vi "8通道控制.vi"() -> ()   [LabVIEW 2010]
uses:
  <vilib>/DAQmx/read.llb/DAQmx Read (Analog 2D DBL NChan NSamp).vi
  <vilib>/DAQmx/read.llb/DAQmx Read (Analog 1D DBL NChan 1Samp).vi
  <vilib>/DAQmx/write.llb/DAQmx Write (Analog 1D DBL NChan 1Samp).vi
  <vilib>/daqmx/miscellaneous.llb/DAQmx Fill In Error Info.vi
panel:
  out "AO overload":bool[](array[boolean])
  in  "啟用控制":bool
  out "速度+加速度":T1(graph)
  out "加速度訊號":T1(graph)
  in  "Kp":dbl[](array[numeric])=[0.0, 0.0, 0.0, 0.0, 0.0, 0.0, 0.0, 0.0]
  in  "Ki":dbl[](array[numeric])=[-500.0, -500.0, -500.0, -500.0, -80.0, -80.0, -80.0, -80.0]
  out "取樣時間誤差(%)":dbl
  out "初始化 input":dbl[][](graph)
  out "速度訊號":T1(graph)
  out "迴圈時間(ms)":dbl
  in  "stop":bool
  out "error out":errorcluster
  in  "ÂoDC®É¶¡(s)":dbl=1.0
  in  "取樣頻率(Hz)":dbl=2000.0
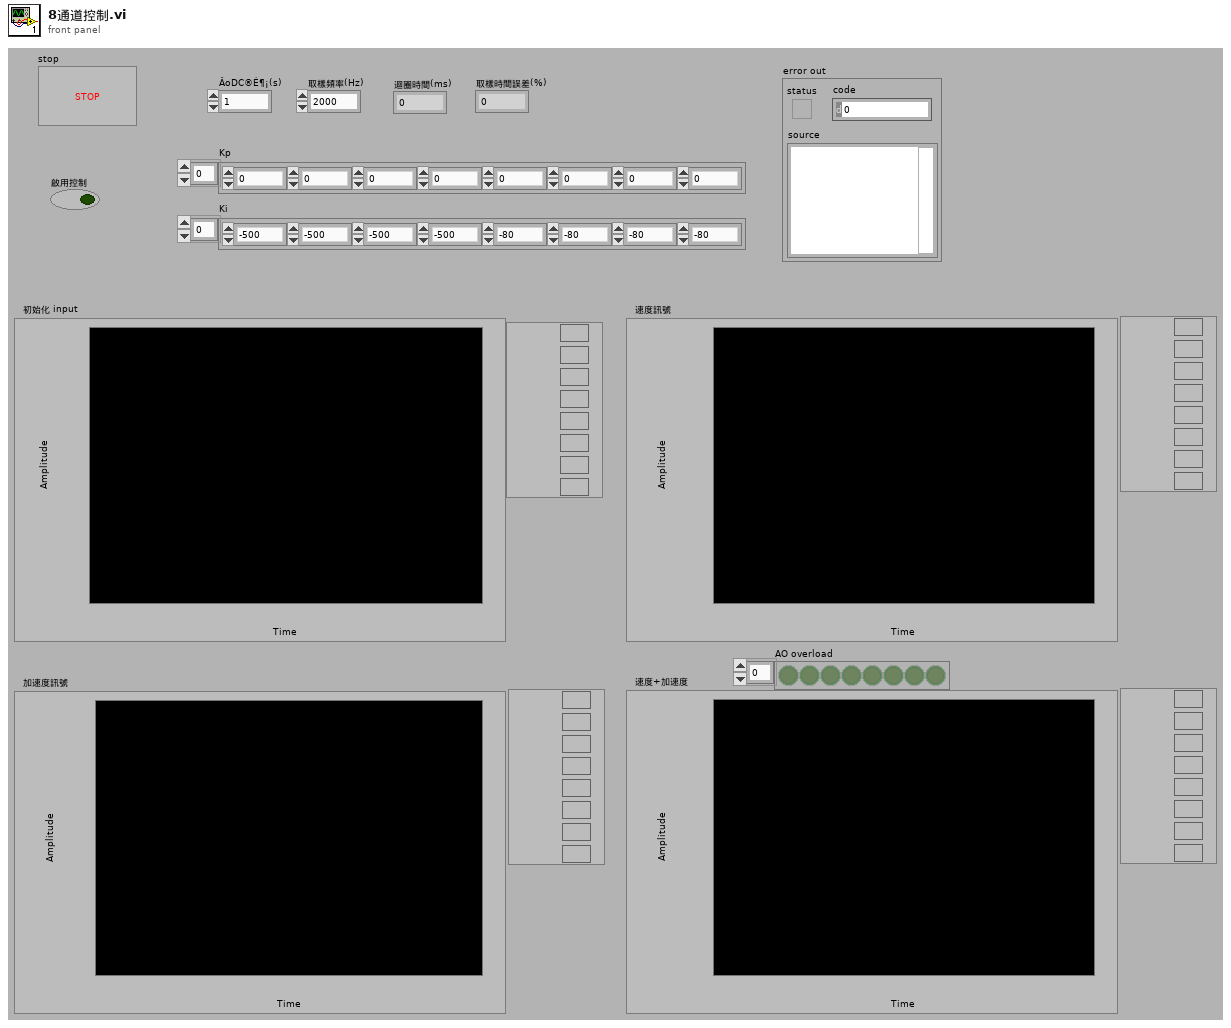
[diagram p1: front panel]
types:
  T1 = cluster{"DC Filter out[0]":dbl, "DC Filter out[1]":dbl, "DC Filter out[2]":dbl, "DC Filter out[3]":dbl, "DC Filter out[4]":dbl, "DC Filter out[5]":dbl, "DC Filter out[6]":dbl, "DC Filter out[7]":dbl}
  T2 = cluster{"[0]":dbl, "[1]":dbl, "[2]":dbl, "[3]":dbl, "[4]":dbl, "[5]":dbl, "[6]":dbl, "[7]":dbl}
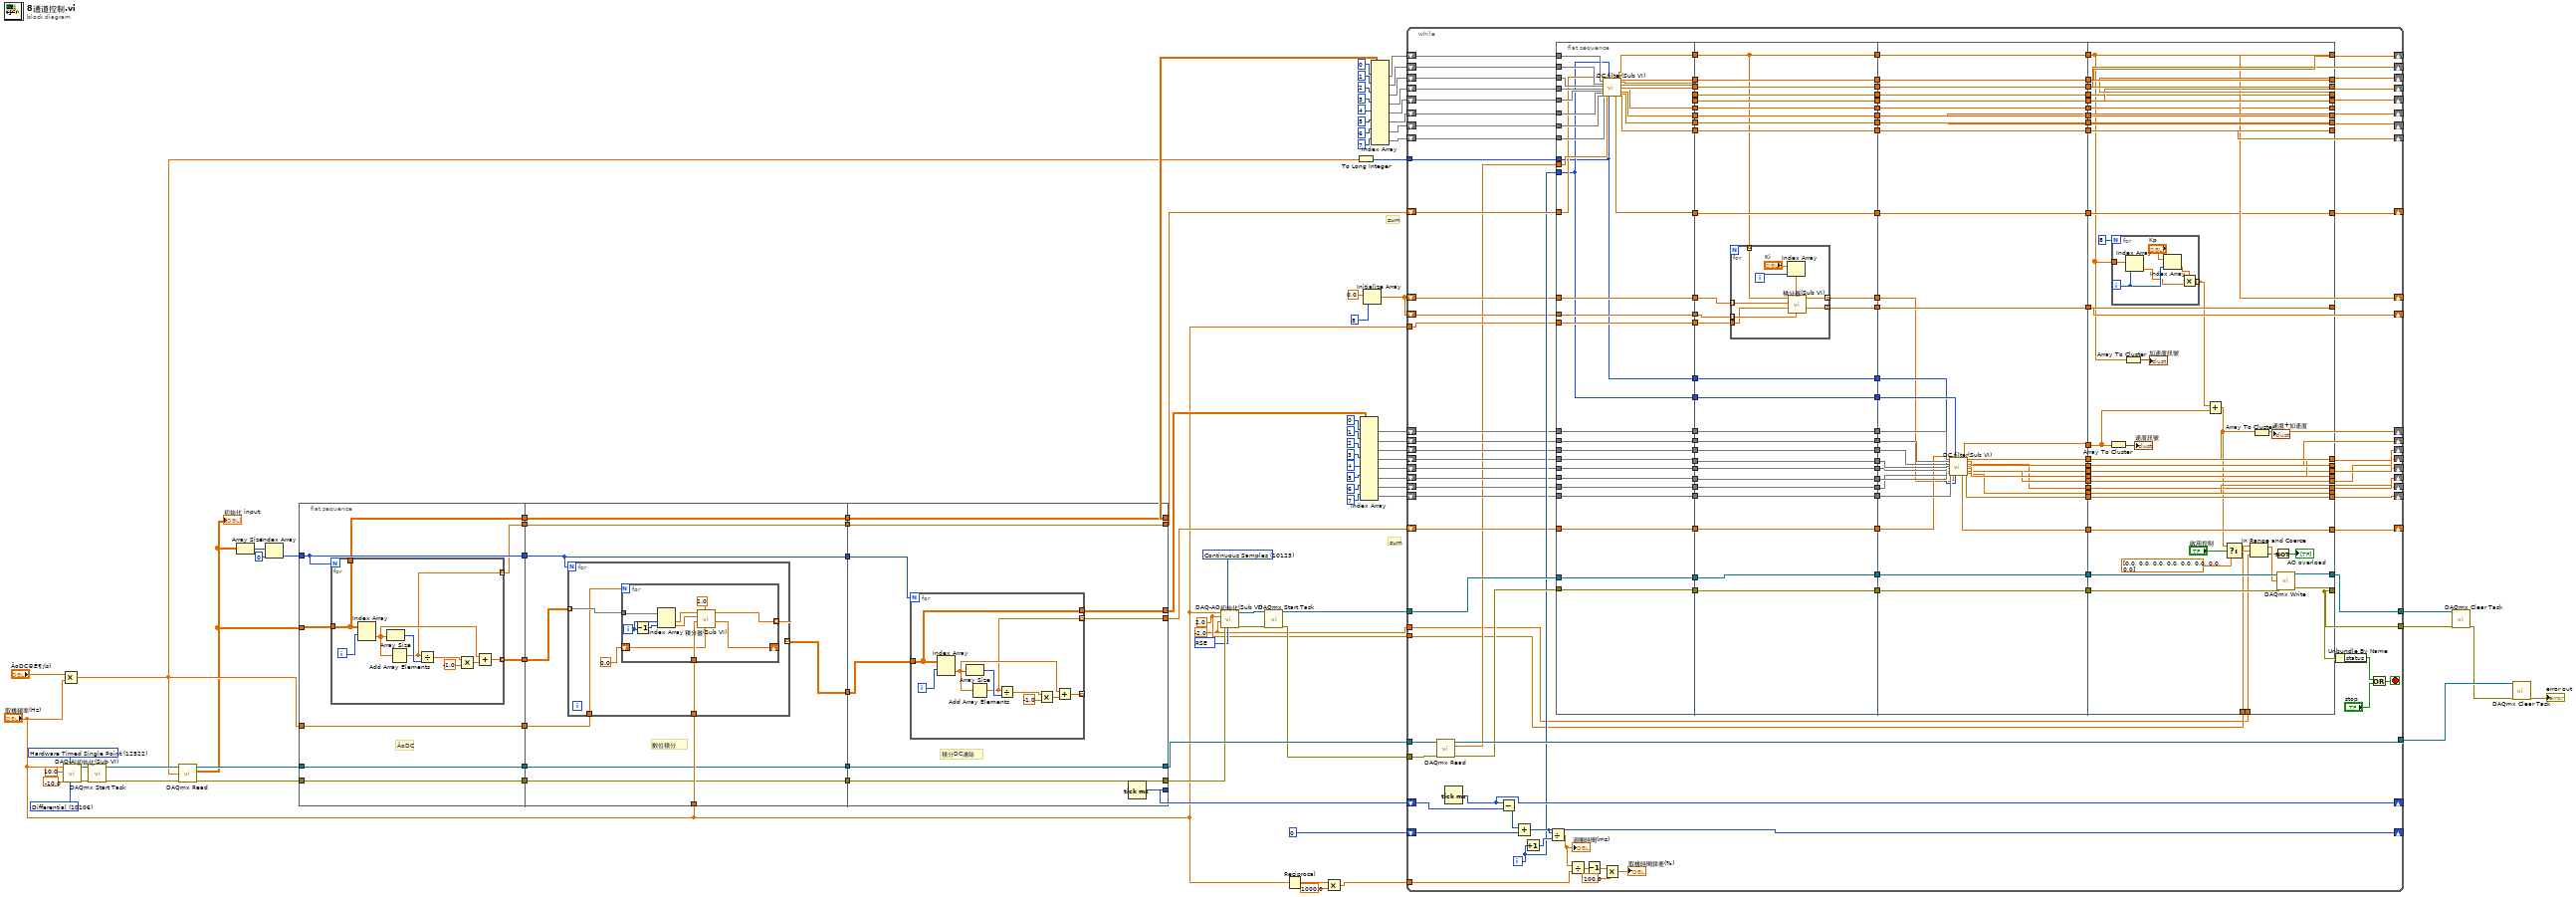
[diagram p0: block diagram]
diagram:
  w7 = 10106 items=["default"=-1, "RSE"=10083, "NRSE"=10078, "Differential"=10106, "Pseudodifferential"=12529] ("input terminal configuration")
  w10 = 10083 items=["Default"=-1, "RSE"=10083, "Differential"=10106, "Pseudodifferential"=12529] ("output terminal configuration")
  w54 = 10123 items=["Finite Samples"=10178, "Continuous Samples"=10123, "Hardware Timed Single Point"=12522] ("sample mode")
  w55 = 12522 items=["Finite Samples"=10178, "Continuous Samples"=10123, "Hardware Timed Single Point"=12522] ("sample mode")
  w1 = -2.0 ("minimum value")
  w2 = 2.0 ("maximum value")
  # "sum"
  # "sum"
  n1 = Multiply(x="ÂoDC®É¶¡(s)", y="取樣頻率(Hz)") -> (x*y=w13:dbl)
  n2 = call "DAQ-AI初始化(Sub VI).vi"("input terminal configuration"=w7, "sample mode"=w55, "minimum value"=-10.0, "maximum value"=10.0, "取樣頻率(Hz)"="取樣頻率(Hz)") -> ("error out"=w87:errorcluster, "task out"=w88:refnum<k21>)  [unwired: 5 in]
  n3 = call <vilib>:"DAQmx Start Task.vi"("task/channels in"=w88, "error in"=w87) -> ("task out"=w90:refnum<k21>, "error out"=w89:errorcluster)  [unwired: 12 in]
  n4 = call-poly <vilib>:"DAQmx Read.vi"("task/channels in"=w90, "number of samples per channel"=w13, "error in"=w89) -> ("task out"=w73:refnum<k21>, "data"=w11:dbl[][], "error out"=w76:errorcluster)  [unwired: 10 in]
  "初始化 input" <- w11
  n5 = Array Size(array=w11) -> (size(s)=w85:i32[])
  n6 = Index Array(array=w85, index=0) -> (element=w83:i32)
  n7 = flat-sequence {
    tunnel: w11 -> [w98]
    tunnel: w83 -> [w96]
    tunnel: [w97] -> w82
    tunnel: [w96] -> w80
    tunnel: w73 -> [w95]
    tunnel: [w95] -> w78
    tunnel: w76 -> [w94]
    tunnel: [w94] -> w75
    tunnel: [w93] -> w70
    tunnel: w13 -> [w93]
    tunnel: [w92] -> w60
    tunnel: [w91] -> w58
    tunnel: w82 -> [w116]
    tunnel: [w115] -> w81
    tunnel: w80 -> [w113]
    tunnel: "取樣頻率(Hz)" -> [w114]
    tunnel: [w113] -> w79
    tunnel: w78 -> [w112]
    tunnel: [w112] -> w77
    tunnel: w75 -> [w111]
    tunnel: [w111] -> w74
    tunnel: w70 -> [w110]
    tunnel: w60 -> [w109]
    tunnel: [w109] -> w59
    tunnel: w58 -> [w108]
    tunnel: [w108] -> w57
    tunnel: w81 -> [w140]
    tunnel: w79 -> [w139]
    tunnel: w77 -> [w138]
    tunnel: w74 -> [w137]
    tunnel: [w138] -> w68
    tunnel: [w137] -> w67
    tunnel: [w136] -> w50
    tunnel: w59 -> [w136]
    tunnel: w57 -> [w135]
    tunnel: [w135] -> w51
    tunnel: [w134] -> w23
    tunnel: [w133] -> w56
    tunnel: [w132] -> w52
    frame #0 {
      # "ÂoDC"
      n8 = for {
        N: w96 -> [_]
        tunnel: w98 -> [w100]
        tunnel: [w102] -> w97 mode=indexing
        tunnel: [w100] -> w92
        tunnel: [w99] -> w91 mode=indexing
        i -> [w103]
        n9 = Index Array(array=w100, index (row)=w103) -> (element=w101:dbl[])  [unwired: 1 in]
        n10 = Array Size(array=w101) -> (size(s)=w104:i32)
        n11 = Add Array Elements(numeric array=w101) -> (sum=w99:dbl)
        n12 = Divide(x=w99, y=w104) -> (x/y=w107:dbl)
        n13 = Multiply(x=w107, y=-1.0) -> (x*y=w106:dbl)
        n14 = Add(x=w101, y=w106) -> (x+y=w102:dbl[])
      }
    }
    frame #1 {
      # "數位積分"
      n15 = for {
        N: w113 -> [_]
        tunnel: w116 -> [w121] mode=indexing
        tunnel: [w120] -> w115 mode=indexing
        tunnel: w110 -> [w119]
        tunnel: w114 -> [w117]
        n16 = for {
          N: w119 -> [_]
          tunnel: w121 -> [w124]
          tunnel: w117 -> [w127]
          shift-right: [w123] -> _
          shift-left: 0.0 ("積分修正量") -> [w125]
          tunnel: [w122] -> w120 mode=indexing
          i -> [w131]
          n17 = Decrement(x=w131) -> (x-1=w130:i32)
          n18 = Index Array(array=w124, index #1=w131, index #2=w130) -> (element #1=w129:dbl, element #2=w128:dbl)
          n19 = call "積分器(Sub VI).vi"("輸入累加ERR回朔"=w125, "I增益"=1.0, "samples (Hz)"=w127, "前一個ERR"=w128, "當下ERR"=w129) -> ("輸出累加ERR回朔"=w123:dbl, "積分修正量"=w122:dbl)  [unwired: 5 in]
        }
      }
    }
    frame #2 {
      # "積分DC濾除"
      n20 = for {
        N: w139 -> [_]
        tunnel: w140 -> [w142]
        tunnel: [w144] -> _ mode=indexing
        tunnel: [w142] -> w134
        tunnel: [w141] -> w133 mode=indexing
        i -> [w145]
        n21 = Index Array(array=w142, index (row)=w145) -> (element=w143:dbl[])  [unwired: 1 in]
        n22 = Array Size(array=w143) -> (size(s)=w146:i32)
        n23 = Add Array Elements(numeric array=w143) -> (sum=w141:dbl)
        n24 = Divide(x=w141, y=w146) -> (x/y=w149:dbl)
        n25 = Multiply(x=w149, y=-1.0) -> (x*y=w148:dbl)
        n26 = Add(x=w143, y=w148) -> (x+y=w144:dbl[])
      }
      n27 = Tick Count (ms)() -> (millisecond timer value=w132:u32)
    }
  }
  n28 = call "DAQ-AO初始化(Sub VI).vi"("output terminal configuration"=w10, "sample mode"=w54, "error in"=w67, "minimum value"=w1, "maximum value"=w2, "取樣頻率(Hz)"="取樣頻率(Hz)") -> ("error out"=w71:errorcluster, "task out"=w72:refnum<k21>)  [unwired: 4 in]
  n29 = call <vilib>:"DAQmx Start Task.vi"("task/channels in"=w72, "error in"=w71) -> ("task out"=w69:refnum<k21>, "error out"=w66:errorcluster)  [unwired: 12 in]
  n30 = Reciprocal(x="取樣頻率(Hz)") -> (1/x=w5:dbl)
  n31 = Multiply(x=w5, y=1000.0) -> (x*y=w4:dbl)
  n32 = To Long Integer(number=w13) -> (32bit integer=w12:i32)
  n33 = Index Array(array=w23, index (row) #1=0, index (row) #2=1, index (row) #3=2, index (row) #4=3, index (row) #5=4, index (row) #6=5, index (row) #7=6, index (row) #8=7) -> (element #1=w22:dbl[], element #2=w21:dbl[], element #3=w20:dbl[], element #4=w19:dbl[], element #5=w18:dbl[], element #6=w17:dbl[], element #7=w16:dbl[], element #8=w15:dbl[])  [unwired: 8 in]
  n34 = Initialize Array(0.0 ("element"), 8 ("dimension size")) -> (w34:dbl[])
  n35 = Index Array(array=w50, index (row) #1=0, index (row) #2=1, index (row) #3=2, index (row) #4=3, index (row) #5=4, index (row) #6=5, index (row) #7=6, index (row) #8=7) -> (element #1=w42:dbl[], element #2=w41:dbl[], element #3=w40:dbl[], element #4=w39:dbl[], element #5=w38:dbl[], element #6=w37:dbl[], element #7=w36:dbl[], element #8=w35:dbl[])  [unwired: 8 in]
  n36 = while {
    tunnel: w69 -> [w282]
    tunnel: w68 -> [w291]
    tunnel: w66 -> [w290]
    tunnel: [w267] -> w65
    tunnel: [w155] -> w63
    tunnel: [w289] -> w64
    shift-right: [w286] -> _
    shift-left: u32 0 -> [w287]
    shift-right: [w283] -> _
    shift-left: w52 -> [w284]
    shift-right: [w255] -> _
    shift-left: w37 -> [w280]
    shift-right: [w249] -> _
    shift-left: w51 -> [w279]
    tunnel: w12 -> [w278]
    shift-right: [w263] -> _
    shift-left: w41 -> [w275]
    shift-right: [w261] -> _
    shift-left: w40 -> [w274]
    shift-right: [w259] -> _
    shift-left: w39 -> [w273]
    shift-right: [w257] -> _
    shift-left: w38 -> [w272]
    shift-right: [w253] -> _
    shift-left: w36 -> [w271]
    shift-right: [w251] -> _
    shift-left: w35 -> [w270]
    shift-right: [w265] -> _
    shift-left: w42 -> [w276]
    shift-right: [w235] -> _
    shift-left: w34 -> [w233]
    shift-right: [w231] -> _
    shift-left: w34 -> [w229]
    tunnel: "取樣頻率(Hz)" -> [w227]
    shift-right: [w164] -> _
    shift-left: w56 -> [w187]
    shift-right: [w180] -> _
    shift-left: w22 -> [w211]
    shift-right: [w178] -> _
    shift-left: w21 -> [w208]
    shift-right: [w176] -> _
    shift-left: w20 -> [w205]
    shift-right: [w174] -> _
    shift-left: w19 -> [w202]
    shift-right: [w172] -> _
    shift-left: w18 -> [w199]
    shift-right: [w170] -> _
    shift-left: w17 -> [w196]
    shift-right: [w168] -> _
    shift-left: w16 -> [w193]
    shift-right: [w166] -> _
    shift-left: w15 -> [w190]
    tunnel: w4 -> [w160]
    tunnel: w2 -> [w151]
    tunnel: w1 -> [w150]
    i -> [w277]
    stop <- w152 stop-if-true
    n37 = call-poly <vilib>:"DAQmx Read.vi"("task/channels in"=w291, "error in"=w290) -> ("task out"=w289:refnum<k21>, "data"=w162:dbl[], "error out"=w281:errorcluster)  [unwired: 11 in]
    n38 = Tick Count (ms)() -> (millisecond timer value=w283:u32)
    n39 = Subtract(x=w283, y=w284) -> (x-y=w288:u32)
    n40 = Add(x=w288, y=w287) -> (x+y=w286:u32)
    n41 = Increment(x=w277) -> (x+1=w285:i32)
    n42 = Divide(x=w286, y=w285) -> (x/y=w161:dbl)
    "迴圈時間(ms)" <- w161
    n43 = flat-sequence {
      tunnel: w282 -> [w327]
      tunnel: [w327] -> w269
      tunnel: w281 -> [w326]
      tunnel: [w326] -> w268
      tunnel: w280 -> [w320]
      tunnel: w279 -> [w308]
      tunnel: w278 -> [w292]
      tunnel: w277 -> [w293]
      tunnel: w162 -> [w309]
      tunnel: w276 -> [w325]
      tunnel: w275 -> [w324]
      tunnel: w274 -> [w323]
      tunnel: w273 -> [w322]
      tunnel: w272 -> [w321]
      tunnel: w271 -> [w319]
      tunnel: w270 -> [w318]
      tunnel: [w317] -> w266
      tunnel: [w316] -> w264
      tunnel: [w315] -> w262
      tunnel: [w314] -> w260
      tunnel: [w313] -> w258
      tunnel: [w312] -> w256
      tunnel: [w311] -> w254
      tunnel: [w310] -> w252
      tunnel: [w307] -> w250
      tunnel: [w306] -> w236
      tunnel: [w305] -> w234
      tunnel: w233 -> [w305]
      tunnel: [w304] -> w230
      tunnel: w229 -> [w304]
      tunnel: [w303] -> w228
      tunnel: w227 -> [w303]
      tunnel: [w302] -> w212
      tunnel: w211 -> [w302]
      tunnel: [w301] -> w209
      tunnel: w208 -> [w301]
      tunnel: [w300] -> w206
      tunnel: w205 -> [w300]
      tunnel: [w299] -> w203
      tunnel: w202 -> [w299]
      tunnel: [w298] -> w200
      tunnel: w199 -> [w298]
      tunnel: [w297] -> w197
      tunnel: w196 -> [w297]
      tunnel: [w296] -> w194
      tunnel: w193 -> [w296]
      tunnel: [w295] -> w191
      tunnel: w190 -> [w295]
      tunnel: [w294] -> w188
      tunnel: w187 -> [w294]
      tunnel: [w293] -> w185
      tunnel: [w292] -> w182
      tunnel: w269 -> [w355]
      tunnel: w268 -> [w354]
      tunnel: w266 -> [w353]
      tunnel: w264 -> [w352]
      tunnel: w262 -> [w351]
      tunnel: w260 -> [w350]
      tunnel: w258 -> [w349]
      tunnel: w256 -> [w348]
      tunnel: w254 -> [w347]
      tunnel: w252 -> [w346]
      tunnel: w250 -> [w345]
      tunnel: [w355] -> w248
      tunnel: [w354] -> w247
      tunnel: [w353] -> w246
      tunnel: [w352] -> w245
      tunnel: [w351] -> w244
      tunnel: [w350] -> w243
      tunnel: [w349] -> w242
      tunnel: [w348] -> w241
      tunnel: [w347] -> w240
      tunnel: [w346] -> w239
      tunnel: [w345] -> w238
      tunnel: [w343] -> w237
      tunnel: w236 -> [w343]
      tunnel: w234 -> [w344]
      tunnel: [w342] -> w232
      tunnel: w230 -> [w341]
      tunnel: w228 -> [w339]
      tunnel: [w340] -> w213
      tunnel: w212 -> [w338]
      tunnel: [w338] -> w210
      tunnel: w209 -> [w337]
      tunnel: [w337] -> w207
      tunnel: w206 -> [w336]
      tunnel: [w336] -> w204
      tunnel: w203 -> [w335]
      tunnel: [w335] -> w201
      tunnel: w200 -> [w334]
      tunnel: [w334] -> w198
      tunnel: w197 -> [w333]
      tunnel: [w333] -> w195
      tunnel: w194 -> [w332]
      tunnel: [w332] -> w192
      tunnel: w191 -> [w331]
      tunnel: [w331] -> w189
      tunnel: w188 -> [w330]
      tunnel: [w330] -> w186
      tunnel: w185 -> [w329]
      tunnel: [w329] -> w184
      tunnel: [w328] -> w183
      tunnel: w182 -> [w328]
      tunnel: w248 -> [w399]
      tunnel: w247 -> [w398]
      tunnel: w246 -> [w397]
      tunnel: w245 -> [w396]
      tunnel: w244 -> [w395]
      tunnel: w243 -> [w394]
      tunnel: w242 -> [w393]
      tunnel: w241 -> [w392]
      tunnel: w240 -> [w391]
      tunnel: w239 -> [w390]
      tunnel: w238 -> [w389]
      tunnel: w237 -> [w388]
      tunnel: w232 -> [w387]
      tunnel: [w399] -> w226
      tunnel: [w398] -> w225
      tunnel: [w397] -> w224
      tunnel: [w396] -> w223
      tunnel: [w395] -> w222
      tunnel: [w394] -> w221
      tunnel: [w393] -> w220
      tunnel: [w392] -> w219
      tunnel: [w391] -> w218
      tunnel: [w390] -> w217
      tunnel: [w389] -> w216
      tunnel: [w388] -> w215
      tunnel: [w387] -> w214
      tunnel: w213 -> [w375]
      tunnel: w210 -> [w386]
      tunnel: w207 -> [w385]
      tunnel: w204 -> [w384]
      tunnel: w201 -> [w383]
      tunnel: w198 -> [w382]
      tunnel: w195 -> [w381]
      tunnel: w192 -> [w380]
      tunnel: w189 -> [w379]
      tunnel: w186 -> [w378]
      tunnel: w184 -> [w377]
      tunnel: w183 -> [w376]
      tunnel: [w374] -> w181
      tunnel: [w373] -> w179
      tunnel: [w372] -> w177
      tunnel: [w371] -> w175
      tunnel: [w370] -> w173
      tunnel: [w369] -> w171
      tunnel: [w368] -> w169
      tunnel: [w367] -> w167
      tunnel: [w366] -> w165
      tunnel: [w365] -> w163
      tunnel: [w429] -> w231
      tunnel: [w409] -> w235
      tunnel: [w430] -> w249
      tunnel: [w431] -> w251
      tunnel: [w432] -> w253
      tunnel: [w433] -> w255
      tunnel: [w434] -> w257
      tunnel: [w435] -> w259
      tunnel: [w436] -> w261
      tunnel: [w437] -> w263
      tunnel: [w438] -> w265
      tunnel: [w425] -> w155
      tunnel: [w427] -> w267
      tunnel: w226 -> [w428]
      tunnel: w225 -> [w426]
      tunnel: w224 -> [w438]
      tunnel: w223 -> [w437]
      tunnel: w222 -> [w436]
      tunnel: w221 -> [w435]
      tunnel: w220 -> [w434]
      tunnel: w219 -> [w433]
      tunnel: w218 -> [w432]
      tunnel: w217 -> [w431]
      tunnel: w216 -> [w430]
      tunnel: w215 -> [w409]
      tunnel: w214 -> [w429]
      tunnel: [w424] -> w180
      tunnel: w181 -> [w424]
      tunnel: [w423] -> w178
      tunnel: w179 -> [w423]
      tunnel: w177 -> [w422]
      tunnel: [w422] -> w176
      tunnel: w175 -> [w421]
      tunnel: [w421] -> w174
      tunnel: w173 -> [w420]
      tunnel: [w420] -> w172
      tunnel: w171 -> [w419]
      tunnel: [w419] -> w170
      tunnel: w169 -> [w418]
      tunnel: [w418] -> w168
      tunnel: w167 -> [w417]
      tunnel: [w417] -> w166
      tunnel: [w416] -> w164
      tunnel: w165 -> [w416]
      tunnel: w163 -> [w413]
      tunnel: w151 -> [w403]
      tunnel: w150 -> [w402]
      frame #0 {
        n44 = call "DC filter(Sub VI).vi"("AI0 input"=w325, "AI1 input"=w324, "AI2 input"=w323, "AI3 input"=w322, "AI4 input"=w321, "AI5 input"=w320, "AI6 input"=w319, "AI7 input"=w318, "sum input (回授)"=w308, "DAQ AI"=w309, "迴圈數"=w293, "ÂoDC°}¦C¤j¤p"=w292) -> ("sum out"=w307:dbl[], "DC Filter out"=w306:dbl[], "AI0 output"=w317:dbl[], "AI1 output"=w316:dbl[], "AI2 output"=w315:dbl[], "AI3 output"=w314:dbl[], "AI4 output"=w313:dbl[], "AI5 output"=w312:dbl[], "AI6 output"=w311:dbl[], "AI7 output"=w310:dbl[])  [unwired: 5 in, 1 out]
      }
      frame #1 {
        n45 = for {
          tunnel: w344 -> [w364] mode=indexing
          tunnel: w343 -> [w363] mode=indexing
          tunnel: [w362] -> w342 mode=indexing
          tunnel: w341 -> [w360] mode=indexing
          tunnel: [w361] -> w340 mode=indexing
          tunnel: w339 -> [w359]
          i -> [w357]
          n46 = Index Array(array="Ki", index=w357) -> (element=w356:dbl)
          n47 = call "積分器(Sub VI).vi"("輸入累加ERR回朔"=w360, "I增益"=w356, "samples (Hz)"=w359, "前一個ERR"=w364, "當下ERR"=w363) -> ("輸出累加ERR回朔"=w362:dbl, "積分修正量"=w361:dbl)  [unwired: 5 in]
        }
      }
      frame #2 {
        n48 = call "DC filter(Sub VI).vi"("AI0 input"=w386, "AI1 input"=w385, "AI2 input"=w384, "AI3 input"=w383, "AI4 input"=w382, "AI5 input"=w381, "AI6 input"=w380, "AI7 input"=w379, "sum input (回授)"=w378, "DAQ AI"=w375, "迴圈數"=w377, "ÂoDC°}¦C¤j¤p"=w376) -> ("sum out"=w366:dbl[], "DC Filter out"=w365:dbl[], "AI0 output"=w374:dbl[], "AI1 output"=w373:dbl[], "AI2 output"=w372:dbl[], "AI3 output"=w371:dbl[], "AI4 output"=w370:dbl[], "AI5 output"=w369:dbl[], "AI6 output"=w368:dbl[], "AI7 output"=w367:dbl[])  [unwired: 5 in, 1 out]
      }
      frame #3 {
        n49 = Array To Cluster(array=w413) -> (cluster=→"速度訊號":T1)
        n50 = for {
          N: 8 -> [_]
          tunnel: w409 -> [w444]
          tunnel: [w439] -> w411 mode=indexing
          i -> [w442]
          n51 = Index Array(array=w444, index=w442) -> (element=w440:dbl)
          n52 = Index Array(array="Kp", index=w442) -> (element=w441:dbl)
          n53 = Multiply(x=w441, y=w440) -> (x*y=w439:dbl)
        }
        n54 = Array To Cluster(array=w409) -> (cluster=→"加速度訊號":T1)
        n55 = Add(x=w411, y=w413) -> (x+y=w407:dbl[])
        n56 = Select(t=w407, s="啟用控制", f=dbl[] [0.0, 0.0, 0.0, 0.0, 0.0, 0.0, 0.0, 0.0]) -> (s? t:f=w405:dbl[])
        n57 = In Range and Coerce(upper limit=w403, x=w405, lower limit=w402) -> (coerced(x)=w404:dbl[], In Range?=w401:bool[])
        n58 = Array To Cluster(array=w407) -> (cluster=→"速度+加速度":T2)
        n59 = Not(x=w401) -> (.not. x?=→"AO overload":bool[])
        n60 = call-poly <vilib>:"DAQmx Write.vi"("task/channels in"=w428, "data"=w404, "error in"=w426) -> ("task out"=w427:refnum<k21>, "error out"=w425:errorcluster)  [unwired: 10 in, 1 out]
      }
    }
    n61 = Divide(x=w161, y=w160) -> (x/y=w159:dbl)
    n62 = Decrement(x=w159) -> (x-1=w158:dbl)
    n63 = Multiply(x=w158, y=100.0) -> (x*y=→"取樣時間誤差(%)":dbl)
    n64 = Unbundle By Name(w155) -> ("status"=w154:bool)
    n65 = Or(x=w154, y="stop") -> (x .or. y?=w152:bool)
  }
  n66 = call <vilib>:"DAQmx Clear Task.vi"("task in"=w65, "error in"=w63) -> ("error out"=w62:errorcluster)  [unwired: 13 in]
  n67 = call <vilib>:"DAQmx Clear Task.vi"("task in"=w64, "error in"=w62) -> ("error out"=→"error out":errorcluster)  [unwired: 13 in]
